vi "Update Service Info.vi"(8 "error in (no error)":errorcluster, 9 "Port":i32, 10 "Type":T1, 11 "DiscoveryService in":refnum<class "NodeDiscovery.lvclass">) -> (0 "error out":errorcluster, 3 "DiscoveryService out":refnum<class "NodeDiscovery.lvclass">)   [LabVIEW 2020, in "Vecto.lvlib" / "NodeDiscovery.lvclass"]
uses:
  NodeDiscovery.lvclass
  proto/ServiceType/Enumeration.ctl
  Update Service Data.ctl
  proto/Service/Data.ctl
  NodeDiscovery.lvclass/NodeDiscovery.ctl
  proto/ServiceType/ServiceType.lvlib
  proto/Service/Service.lvlib
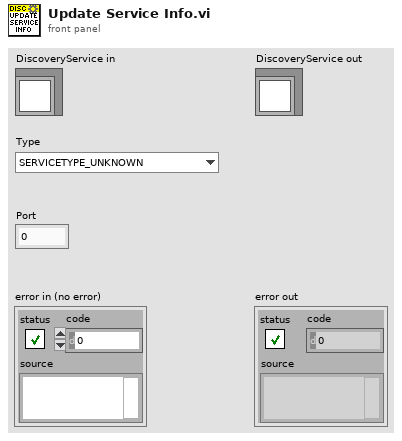
[diagram p1: front panel]
types:
  T1 = typedef "ServiceType.lvlib/Enumeration.ctl" = enum16{"SERVICETYPE_UNKNOWN", "SERVICETYPE_TCPSERVER", "SERVICETYPE_HTTPSERVER"}
  T2 = typedef "Vecto.lvlib/NodeDiscovery.lvclass/Update Service Data.ctl" = cluster{"Service":T3}
  T3 = typedef "Service.lvlib/Data.ctl" = cluster{"type":T1, "port":i32}
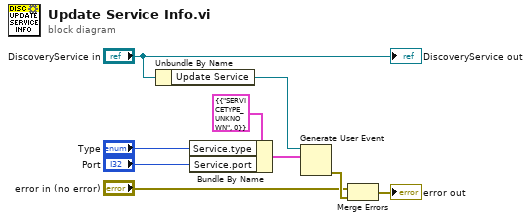
[diagram p0: block diagram]
diagram:
  n1 = Unbundle By Name("DiscoveryService in") -> ("Update Service"=w9:refnum<user-event>)
  n2 = Bundle By Name(cluster=T2 {"Service"={"type"=enum."SERVICETYPE_UNKNOWN", "port"=0}} ("event data"), "Service.type"="Type", "Service.port"="Port") -> (w7:T2)
  n3 = Generate User Event(user event=w9, event data cluster=w7) -> (error out=w6:errorcluster)  [unwired: 2 in, 1 out]
  n4 = Merge Errors("error in (no error)", w6) -> (→"error out":errorcluster)
  "DiscoveryService out" <- "DiscoveryService in"
